vi "mxwScript_API_Option_ErrorDialog.vi"(8 "error in (no error)":errorcluster, 10 "show?":bool, 11 "options in":T1[](array[typedef])) -> (0 "error out":errorcluster, 3 "options out":T1[](array[typedef]))   [LabVIEW 2017]
uses:
  codeGenAPISupport.llb/cgAPI_mxwScript_OptionData.ctl
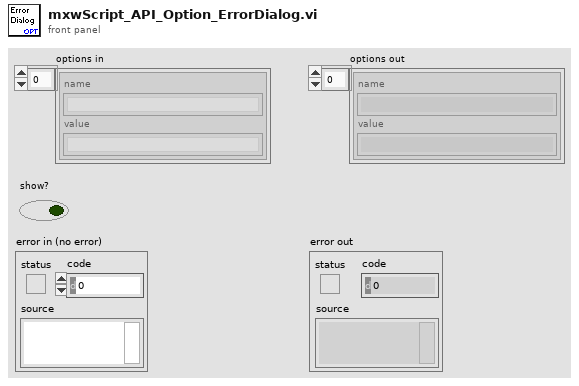
[diagram p1: front panel]
types:
  T1 = typedef "cgAPI_mxwScript_OptionData.ctl" = cluster{"name":string, "value":string}
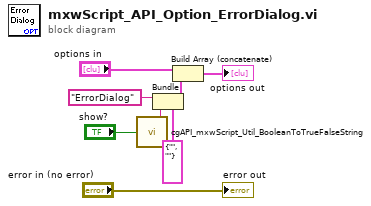
[diagram p0: block diagram]
diagram:
  n1 = call "cgAPI_mxwScript_Util_BooleanToTrueFalseString.vi"("boolean"="show?") -> ("TRUE/FALSE text"=w1:string)  [unwired: 4 out]
  n2 = Bundle(cluster=T1 {"name"="", "value"=""} ("optionData"), "name"="ErrorDialog", "value"=w1) -> (w6:T1)
  n3 = Build Array (concatenate)("options in", w6) -> (→"options out":T1[])
  "error out" <- "error in (no error)"
